vi "Demo_Andon Datetime string array to Timestamp.vi"(8 "error in (no error)":errorcluster, 10 "String Array In":string[][](array[string])) -> (0 "error out":errorcluster, 2 "Time Stamp Out":timestamp[](array[timestamp]) format="%<%X>T")   [LabVIEW 2017]
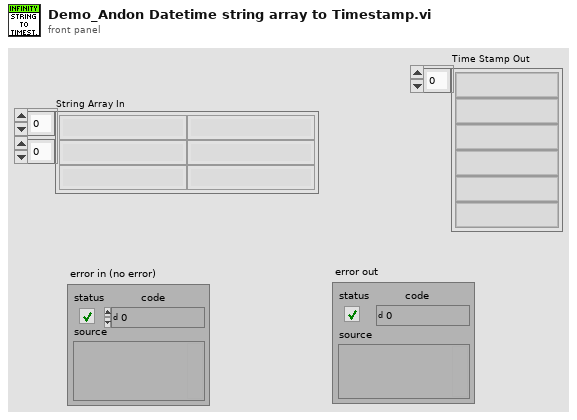
[diagram p1: front panel]
types:
  T1 = cluster{"second":i32, "minute":i32, "hour":i32, "day of month":i32, "month":i32, "year":i32, "day of week":i32, "day of year":i32, "is DST":i32}
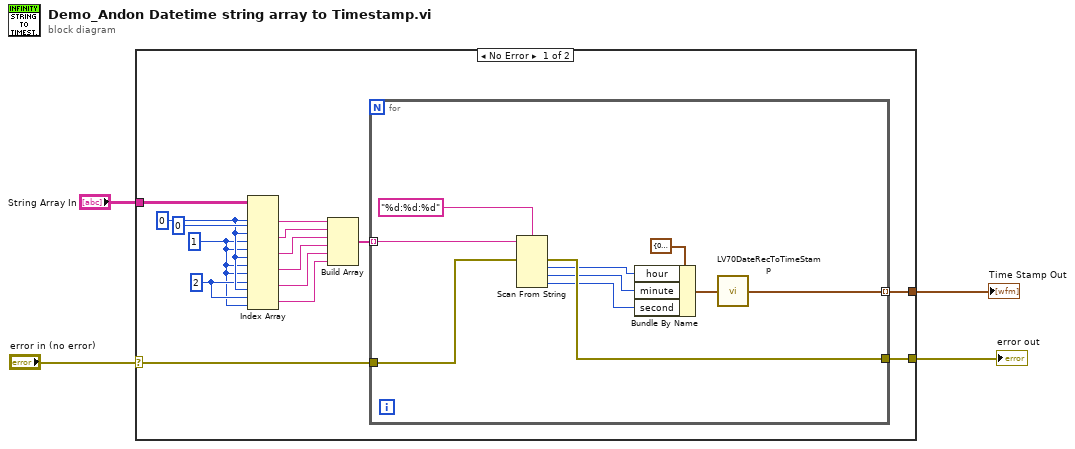
[diagram p0: block diagram]
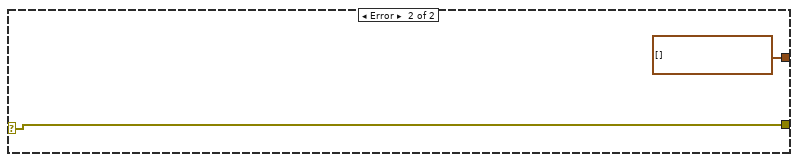
[diagram p2: hidden frame]
diagram:
  n1 = case shown="No Error" "error in (no error)" {
    selector: "error in (no error)" -> [w6 w31]
    tunnel: "String Array In" -> [w18 _]
    tunnel: [w8 timestamp[] []] -> w3
    tunnel: [w5 w31] -> w1
    frame No Error {
      w16 = 2 ("disabled index (col)")
      w15 = 1 ("disabled index (col)")
      w17 = 0 ("index (row)")
      n2 = Index Array(array=w18, index (row) #1=w17, index (col) #1=0 ("disabled index (col)"), index (row) #2=w17, index (col) #2=w15, index (row) #3=w15, index (col) #3=w17, index (row) #4=w15, index (col) #4=w15, index (row) #5=w16, index (col) #5=w17, index (row) #6=w16, index (col) #6=w15) -> (element #1=w14:string, element #2=w13:string, element #3=w12:string, element #4=w11:string, element #5=w10:string, element #6=w7:string)
      n3 = Build Array(w14, w13, w12, w11, w10, w7) -> (w9:string[])
      n4 = for {
        tunnel: w9 -> [w26] mode=indexing
        tunnel: [w25] -> w8 mode=indexing
        tunnel: w6 -> [w24]
        tunnel: [w23] -> w5
        n5 = Scan From String(format string="%d:%d:%d", input string=w26, error in=w24) -> (error out=w23:errorcluster, output 1=w22:i32, output 2=w21:i32, output 3=w20:i32)  [unwired: 4 in, 2 out]
        n6 = Bundle By Name(cluster=T1 {"second"=0, "minute"=0, "hour"=0, "day of month"=1, "month"=1, "year"=2018, "day of week"=0, "day of year"=0, "is DST"=0} ("date time rec"), "hour"=w22, "minute"=w21, "second"=w20) -> (w28:T1)
        n7 = call <vilib>:"LV70DateRecToTimeStamp.vi"("date time rec"=w28) -> ("Time Stamp"=w25:timestamp)
      }
    }
    frame Error {
    }
  }
  "Time Stamp Out" <- w3
  "error out" <- w1
